vi "getExceptionMessage.vi"(9 "exception":i32, 11 "Job.StaticVIRef in":refnum<class "Job.StaticVIRef.lvclass">) -> (0 "exception message":string, 1 "exception dup":i32, 3 "warning?":bool)   [LabVIEW 2013, in "openCronJob.lvlib" / "Job.StaticVIRef.lvclass"]
uses:
  Job.StaticVIRef.lvclass
  Job/Job.lvclass
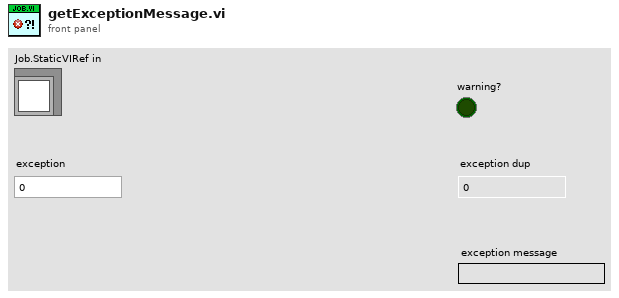
[diagram p1: front panel]
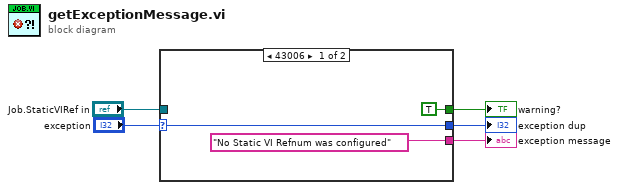
[diagram p0: block diagram]
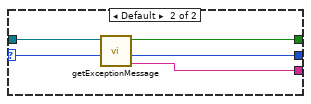
[diagram p2: hidden frame]
diagram:
  n1 = case shown="43006" "exception" {
    selector: "exception" -> [w8 w9]
    tunnel: ["No Static VI Refnum was configured" ("format string") w13] -> w5
    tunnel: [w8 w12] -> w4
    tunnel: [TRUE ("warning?") w11] -> w3
    tunnel: "Job.StaticVIRef in" -> [_ w10]
    frame 43006 {
    }
    frame Default {
      n2 = call-parent "getExceptionMessage.vi"("exception"=w9, "Job in"=w10) -> ("exception message"=w13:string, "exception dup"=w12:i32, "warning?"=w11:bool)  [unwired: 7 in]
    }
  }
  "exception dup" <- w4
  "exception message" <- w5
  "warning?" <- w3
